vi "Robot Main.vi"() -> ()   [LabVIEW 2013]
doc: "This VI imlements the framework and scheduler for your robotics program. It should not be necessary to modify the framework. You are expected to add your code to the VIs called from Robot Main, the ones located in the Team Code within the project."
uses:
  <vilib>/Rock Robotics/SystemInterfaces/DIO/FPGA_DIOChannel.ctl
panel:
  in  "PWM Rate (Hz)":sgl=1000.0
  in  "DIO Blue":T1=enum."DIO 2"
  in  "DIO Green":T1
  in  "DIO Red":T1=enum."DIO 3"
  in  "Max Duty Cycle":sgl=0.4
  in  "Finish":bool
  out "Color":u32(colorbox)
  in  "Value":dbl(slide) scale=0.0..1.0
  in  "Saturation":dbl(slide) scale=0.0..1.0
  in  "Speed":dbl=1.0 format="%#_13g"
  in  "R":u8(slide) scale=0.0..255.0
  in  "G":u8(slide) scale=0.0..255.0
  in  "B":u8(slide) scale=0.0..255.0
  in  "Mood":bool caption="Mood Lights?"
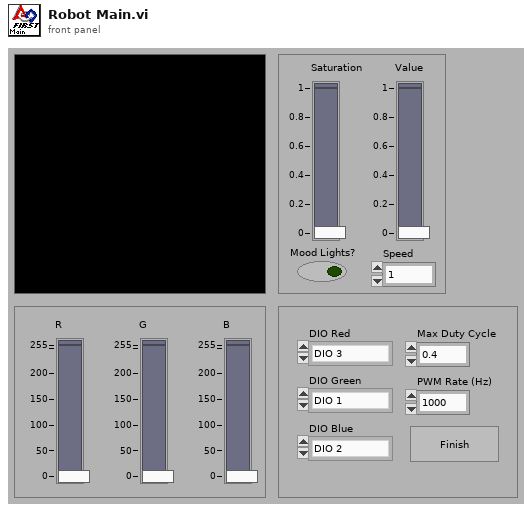
[diagram p1: front panel]
types:
  T1 = typedef "FPGA_DIOChannel.ctl" = enum8{"DIO 1", "DIO 2", "DIO 3", "DIO 4", "DIO 5", "DIO 6", "DIO 7", "DIO 8", "DIO 9", "DIO 10", "DIO 11", "DIO 12", "DIO 13", "DIO 14", "Invalid"}
  T2 = typedef "LEDStripRef.ctl" = cluster{"PWM Rate (Hz)":sgl, "Max Duty Cycle":sgl, "DigitalOutputRed":T3, "DigitalOutputGreen":T3, "DigitalOutputBlue":T3, "DevStatus":errorcluster}
  T3 = typedef "WPI_DigitalOutputDevRef.ctl" = cluster{"Digital Module":T4, "DIO Channel":T1, "DevStatus":errorcluster}
  T4 = typedef "FPGA_TypedefDigitalModule.ctl" = enum16{"Digital Module 1", "Digital Module 2"}
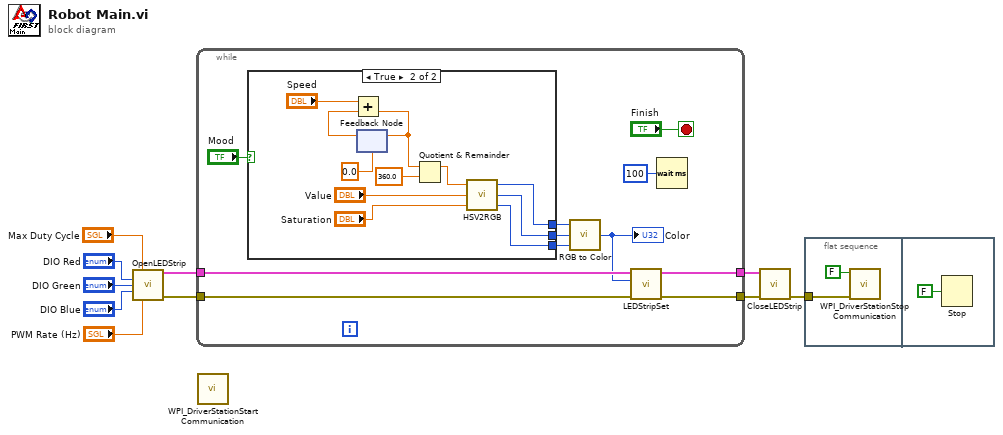
[diagram p0: block diagram]
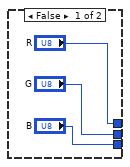
[diagram p2: hidden frame]
diagram:
  n1 = call "OpenLEDStrip.vi"("Max Duty Cycle (1)"="Max Duty Cycle", "DIO Channel Red"="DIO Red", "DIO Channel Green"="DIO Green", "DIO Channel Blue"="DIO Blue", "PWM Rate (Hz)"="PWM Rate (Hz)") -> ("LEDStripRef"=w5:T2, "error out"=w4:errorcluster)  [unwired: 9 in]
  n2 = while {
    tunnel: w5 -> [w19]
    tunnel: w4 -> [w18]
    tunnel: [w12] -> w3
    tunnel: [w11] -> w2
    stop <- "Finish" stop-if-true
    n3 = case shown="True" "Mood" {
      tunnel: ["R" w27] -> w16
      tunnel: ["G" w26] -> w15
      tunnel: ["B" w25] -> w14
      frame False {
      }
      frame True {
        n4 = feedback #1(0.0) -> (w32:dbl)
        n5 = Add(x="Speed", y=w32) -> (x+y=w30:dbl)
        n6 = feedback-in #1(w30) -> ()
        n7 = Quotient & Remainder(x=w30, y=360.0) -> (x-y*floor(x/y)=w28:dbl)  [unwired: 1 out]
        n8 = call "HSV2RGB.vi"("Value"="Saturation", "Saturation"="Value", "Hue"=w28) -> ("Blue"=w25:u8, "Green"=w26:u8, "Red"=w27:u8)
      }
    }
    n9 = call <vilib>:"RGB to Color.vi"("B"=w14, "G"=w15, "R"=w16) -> ("Color"=w17:u32)
    "Color" <- w17
    n10 = call "LEDStripSet.vi"("error in"=w18, "Color"=w17, "LEDStripRef in"=w19) -> ("error out"=w11:errorcluster, "LEDStripRef out"=w12:T2)  [unwired: 7 in]
    n11 = Wait (ms)(milliseconds to wait=u32 100) -> ()  [unwired: 1 out]
  }
  n12 = call <vilib>:"WPI_DriverStationStart Communication.vi"() -> ()  [unwired: 1 in, 11 out]
  n13 = call "CloseLEDStrip.vi"("error in (no error)"=w2, "LEDStripRef in"=w3) -> ("error out"=w1:errorcluster)  [unwired: 9 in]
  n14 = flat-sequence {
    tunnel: w1 -> [w37]
    frame #0 {
      n15 = call <vilib>:"WPI_DriverStationStop Communication.vi"("error in (no error)"=w37, "StopCommunication"=FALSE) -> ()  [unwired: 9 in, 1 out]
    }
    frame #1 {
      n16 = Stop(stop? (T)=FALSE) -> ()
    }
  }
